vi "Interface.vi"() -> ()   [LabVIEW 2019, in "Error Interface.lvclass"]
uses:
  Error Interface.lvclass
  Robot/Universal Robot/Universal Robot.lvclass
  C:/_Code/Development/Sub-Zero Functional Test/standard hardware/Universal Robots/UR LabVIEW Interface/Classes/Application/Application Interfaces/Application Interface/Application Interface.lvclass
  ErrorEvent.ctl
  Error Interface.lvclass/Error Interface.ctl
  Application.lvclass
panel:
  in  "Clear Log":bool
  in  "Download Log":bool
  in  "Error Log":i32(listbox)
  in  "interface":refnum<class "Error Interface.lvclass">
  in  "robot":refnum<class "Universal Robot.lvclass">
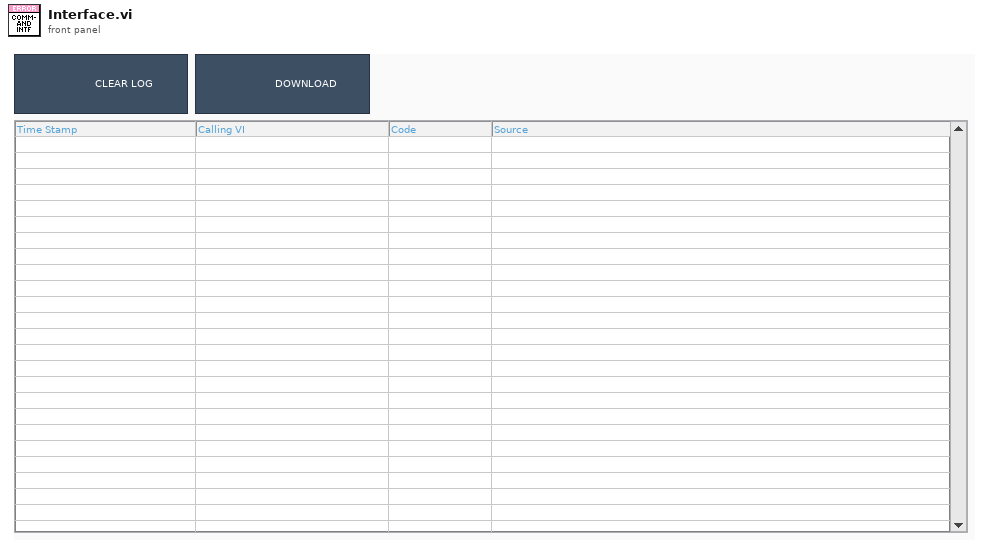
[diagram p1: front panel]
types:
  T1 = typedef "Application.lvclass/ErrorEvent.ctl" = cluster{"VI":string, "Time Stamp":timestamp, "Error":errorcluster, "Fatal":bool}
  T2 = typedef "Application.lvclass/FrontPanelControls.ctl" = cluster{"Operation Interface":refnum<vi>, "Program Interface":refnum<vi>, "Command Interface":refnum<vi>, "Socket Interface":refnum<vi>, "Error Interface":refnum<vi>}
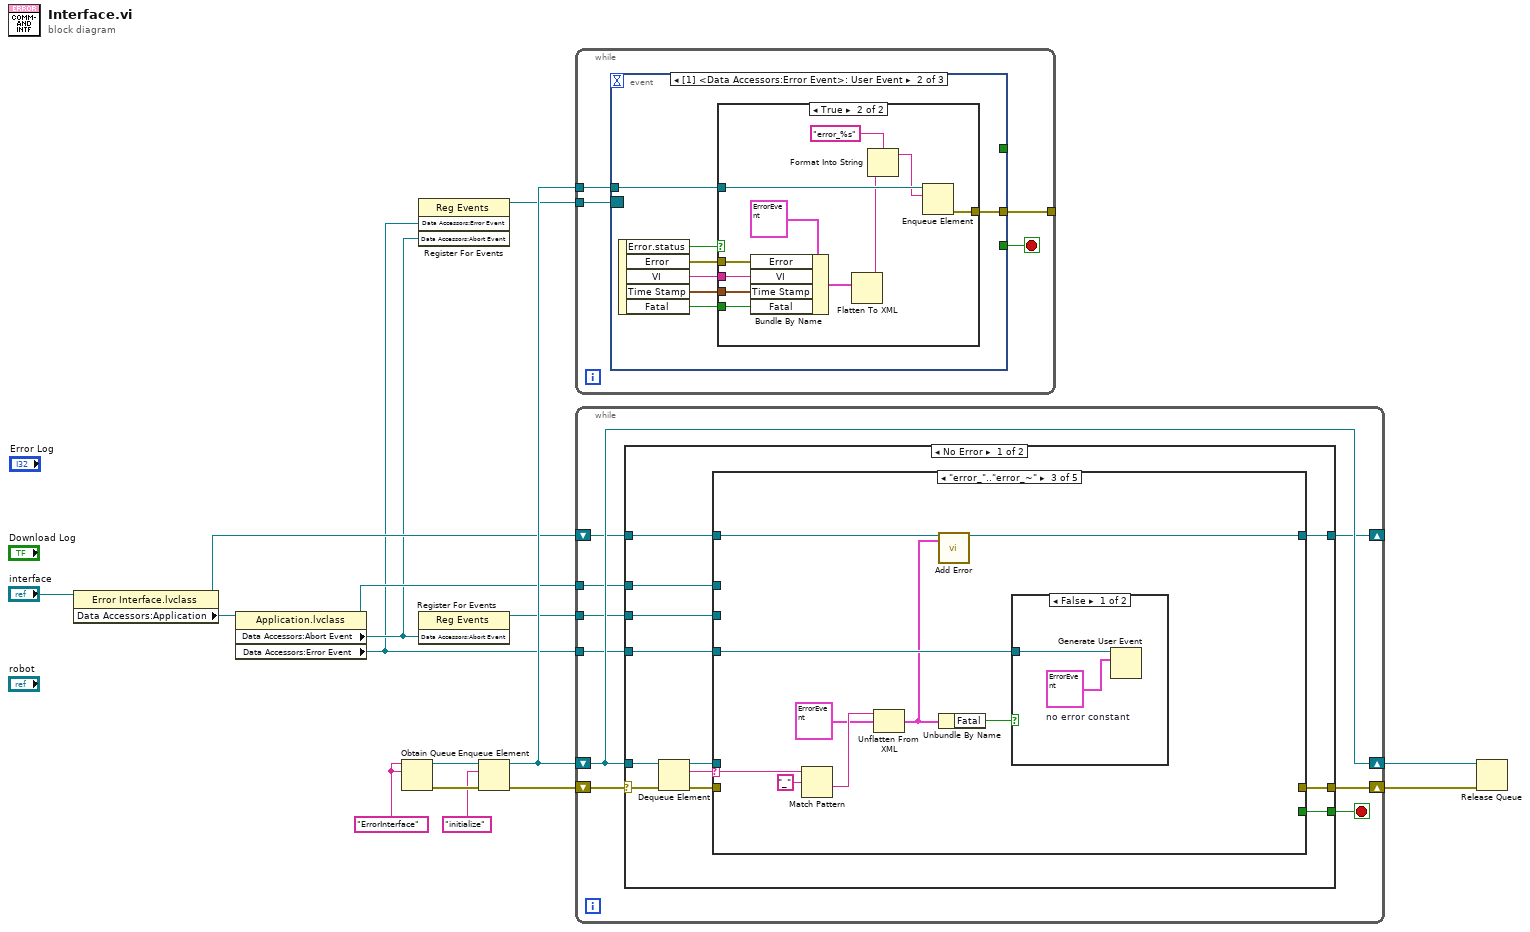
[diagram p0: block diagram]
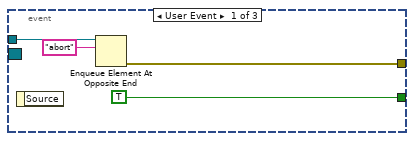
[diagram p2: hidden frame]
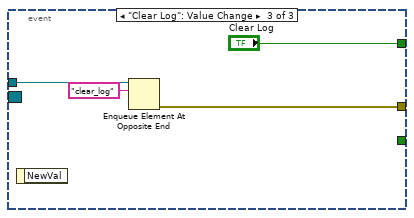
[diagram p4: hidden frame]
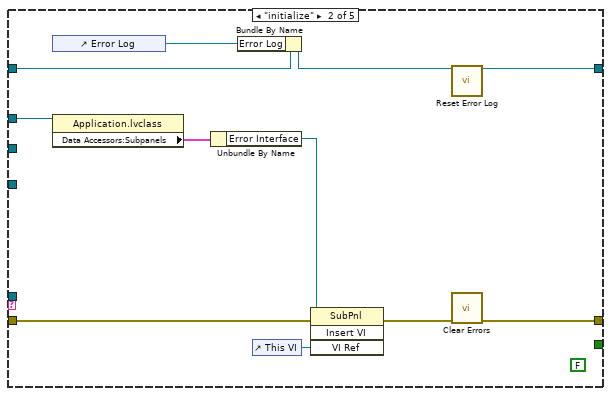
[diagram p6: hidden frame]
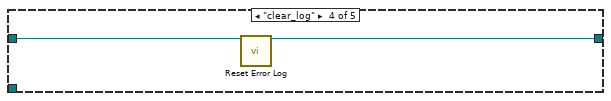
[diagram p8: hidden frame]
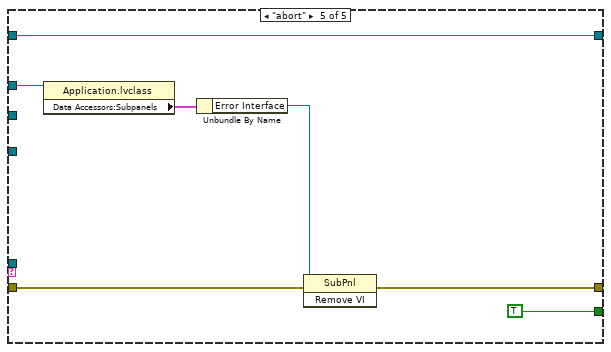
[diagram p9: hidden frame]
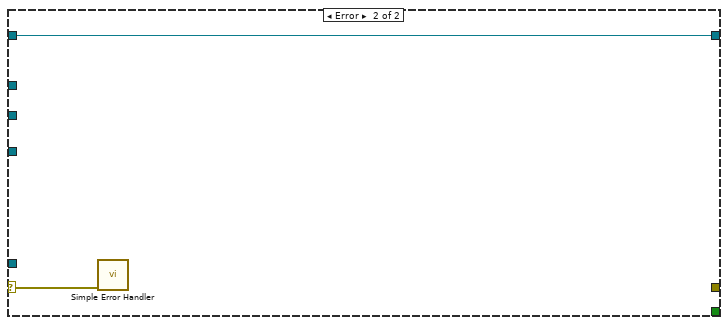
[diagram p10: hidden frame]
diagram:
  w11 = "ErrorInterface" ("name (unnamed)")
  n1 = property class="Error Interface.lvclass"(reference="interface") -> (reference out=w6:refnum<class "Error Interface.lvclass">, "Data Accessors:Application"=w8:refnum<class "Application.lvclass">)  [unwired: 1 in, 1 out]
  n2 = property class="Application.lvclass"(reference=w8) -> (reference out=w5:refnum<class "Application.lvclass">, "Data Accessors:Abort Event"=w2:refnum<user-event>, "Data Accessors:Error Event"=w1:refnum<user-event>)  [unwired: 1 in, 1 out]
  n3 = Obtain Queue(name (unnamed)=w11, element data type=w11) -> (queue out=w15:refnum<queue>, error out=w16:errorcluster)  [unwired: 3 in, 1 out]
  n4 = register-events(w1, w2) -> (reference out=w3:refnum<event-registration>)  [unwired: 2 in, 1 out]
  n5 = register-events(w2) -> (reference out=w4:refnum<event-registration>)  [unwired: 2 in, 1 out]
  n6 = Enqueue Element(queue=w15, element="initialize", error in (no error)=w16) -> (queue out=w12:refnum<queue>, error out=w13:errorcluster)  [unwired: 1 in, 1 out]
  n7 = while {
    tunnel: w12 -> [w20]
    tunnel: w3 -> [w19]
    tunnel: [w18] -> _
    stop <- w17 stop-if-true
    n8 = event shown="[1] <Data Accessors:Error Event>: User Event" {
      selector: w19 -> [_ _ _]
      dyn-events: _ -> [_ _ _]
      timeout: _ -> [_ _ _]
      tunnel: w20 -> [w24 w31 w45]
      tunnel: [w23 w30 w44] -> w18
      tunnel: [TRUE _ _] -> w17
      tunnel: [_ _ "Clear Log"] -> _
      event User Event {
        n9 = event-data() -> ()  [unwired: 1 in, 1 out]
        n10 = Enqueue Element At Opposite End(queue=w24, element="abort") -> (error out=w23:errorcluster)  [unwired: 2 in, 2 out]
      }
      event User Event {
        n11 = event-data() -> ("Error.status"=w29:bool, "Error"=w28:errorcluster, "VI"=w27:string, "Time Stamp"=w26:timestamp, "Fatal"=w25:bool)  [unwired: 1 in]
        n12 = case shown="True" w29 {
          tunnel: w28 -> [_ w42]
          tunnel: w27 -> [_ w41]
          tunnel: w31 -> [_ w39]
          tunnel: [_ w38] -> w30
          tunnel: w26 -> [_ w33]
          tunnel: w25 -> [_ w32]
          frame False {
          }
          frame True {
            n13 = Bundle By Name(cluster=T1 {"VI"="", "Time Stamp"=timestamp(0 s since 1904-01-01), "Error"={"status"=FALSE, "code"=0, "source"=""}, "Fatal"=FALSE} ("Error"), "Error"=w42, "VI"=w41, "Time Stamp"=w33, "Fatal"=w32) -> (w40:T1)
            n14 = Flatten To XML(anything=w40) -> (xml string=w37:string)
            n15 = Format Into String(format string="error_%s", w37) -> (resulting string=w36:string)  [unwired: 2 in, 1 out]
            n16 = Enqueue Element(queue=w39, element=w36) -> (error out=w38:errorcluster)  [unwired: 2 in, 2 out]
          }
        }
      }
      event "Clear Log": Value Change {
        n17 = event-data() -> ()  [unwired: 1 in, 1 out]
        n18 = Enqueue Element At Opposite End(queue=w45, element="clear_log") -> (error out=w44:errorcluster)  [unwired: 2 in, 2 out]
      }
    }
  }
  n19 = while {
    shift-right: [w53] -> w9
    shift-left: w13 -> [w55]
    shift-right: [w54] -> w10
    shift-left: w12 -> [w54]
    tunnel: w1 -> [w51]
    tunnel: w4 -> [w50]
    shift-right: [w48] -> _
    shift-left: w6 -> [w49]
    tunnel: w5 -> [w47]
    stop <- w52 stop-if-true
    n20 = case shown="No Error" w55 {
      selector: w55 -> [w66 w101]
      tunnel: w54 -> [w67 _]
      tunnel: [w62 _] -> w53
      tunnel: [w61 _] -> w52
      tunnel: w51 -> [w60 _]
      tunnel: w50 -> [w59 _]
      tunnel: w49 -> [w58 w102]
      tunnel: [w57 w102] -> w48
      tunnel: w47 -> [w56 _]
      frame No Error {
        n21 = Dequeue Element(queue=w67, error in (no error)=w66) -> (queue out=w63:refnum<queue>, element=w64:string, error out=w65:errorcluster)  [unwired: 1 in, 1 out]
        n22 = case shown="\"error_\"..\"error_~\"" w64 {
          selector: w64 -> [_ _ w87 _ _]
          tunnel: w65 -> [w69 w71 _ _ w99]
          tunnel: w63 -> [_ _ _ _ _]
          tunnel: [w69 w72 _ _ w98] -> w62
          tunnel: [_ _ _ _ TRUE] -> w61
          tunnel: w60 -> [_ _ w84 _ _]
          tunnel: w59 -> [_ _ _ _ _]
          tunnel: w58 -> [w68 w77 w82 w93 w95]
          tunnel: [w68 w76 w81 w92 w95] -> w57
          tunnel: w56 -> [_ w74 _ _ w94]
          frame Default {
          }
          frame "initialize" {
            (unwired) FALSE ("Running")
            n23 = control-ref of="Error Log"() -> (w70:refnum<vi>)
            n24 = property class="Application.lvclass"(reference=w74) -> ("Data Accessors:Subpanels"=w79:T2)  [unwired: 1 in, 2 out]
            n25 = Unbundle By Name(w79) -> ("Error Interface"=w78:refnum<vi>)
            n26 = Bundle By Name(cluster=w77, "Error Log"=w70) -> (w75:refnum<class "Error Interface.lvclass">)
            n27 = control-ref of="This VI"() -> (w80:refnum<vi>)
            n28 = invoke class="SubPnl" method="Insert VI"(reference=w78, error in=w71, "VI Ref"=w80) -> (error out=w73:errorcluster)  [unwired: 1 in, 3 out]
            n29 = call "Reset Error Log.vi"("Socket Auto Connect in"=w75) -> ("Socket Auto Connect out"=w76:refnum<class "Error Interface.lvclass">)  [unwired: 17 in, 1 out]
            n30 = call <vilib>:"Clear Errors.vi"("error in (no error)"=w73) -> ("error out"=w72:errorcluster)  [unwired: 5 in, 1 out]
          }
          frame "error_".."error_~" {
            n31 = Match Pattern(string=w87, regular expression="_") -> (after substring=w89:string)  [unwired: 1 in, 3 out]
            n32 = Unflatten From XML(xml string=w89, type=T1 {"VI"="", "Time Stamp"=timestamp(0 s since 1904-01-01), "Error"={"status"=FALSE, "code"=0, "source"=""}, "Fatal"=FALSE} ("Error")) -> (value=w83:T1)  [unwired: 1 in, 1 out]
            n33 = call "Add Error.vi"("Error Interface In"=w82, "Error"=w83) -> ("Error Interface Out"=w81:refnum<class "Error Interface.lvclass">)  [unwired: 16 in, 1 out]
            n34 = Unbundle By Name(w83) -> ("Fatal"=w85:bool)
            n35 = case shown="False" w85 {
              tunnel: w84 -> [w91 _]
              frame False {
                w90 = T1 {"VI"="", "Time Stamp"=timestamp(0 s since 1904-01-01), "Error"={"status"=FALSE, "code"=0, "source"=""}, "Fatal"=FALSE}  # no error constant
                n36 = Generate User Event(user event=w91, event data cluster=w90) -> ()  [unwired: 2 in, 2 out]
              }
              frame True {
              }
            }
          }
          frame "clear_log" {
            n37 = call "Reset Error Log.vi"("Socket Auto Connect in"=w93) -> ("Socket Auto Connect out"=w92:refnum<class "Error Interface.lvclass">)  [unwired: 17 in, 1 out]
          }
          frame "abort" {
            n38 = property class="Application.lvclass"(reference=w94) -> ("Data Accessors:Subpanels"=w97:T2)  [unwired: 1 in, 2 out]
            n39 = Unbundle By Name(w97) -> ("Error Interface"=w96:refnum<vi>)
            n40 = invoke class="SubPnl" method="Remove VI"(reference=w96, error in=w99) -> (error out=w98:errorcluster)  [unwired: 1 in, 2 out]
          }
        }
      }
      frame Error {
        n41 = call <vilib>:"Simple Error Handler.vi"("error in (no error)"=w101) -> ()  [unwired: 4 in, 5 out]
      }
    }
  }
  n42 = Release Queue(queue=w10, error in (no error)=w9) -> ()  [unwired: 1 in, 3 out]
